vi "Demo_PlotMusic_app.vi"   [LabVIEW 2021, in "RocketPlotDemo.lvlib"]
uses:
  Demo/RocketPlotDemo.lvlib
  Classes/RocketPlotHandle/SubVIs/Init Options.ctl
  TypeDefs/TimeZone.ctl
  TypeDefs/plot load data V2.ctl
  TypeDefs/plot properties V2.ctl
  TypeDefs/plot attributes V2.ctl
  TypeDefs/Plot scale axis properties.ctl
  TypeDefs/Plot general properties.ctl
  <vilib>/sound2/lvsound2.llb/Sampling Mode.ctl
  Classes/RocketPlotPanel/RocketPlotPanel.lvclass/RocketPlotPanel.ctl
  Classes/BjusticePlotHandle/BjusticePlotHandle.lvclass/BjusticePlotHandle.ctl
  4dfea61d-788a-4186-b191-4cde70d6fed2.vi
  966c8643-725a-46bd-9dd0-b91467cf4ddd.vi
  eb0507fd-03f2-4275-8513-22fa9a77d05c.vi
  2cc444ce-eb93-4e53-95b9-bbf802b1ec09.vi
  44d01159-0067-4c41-b020-b8d23d8c44ab.vi
  0323ff41-b8ad-4ed8-8c31-07cadd3001fa.vi
  286f873d-ace6-4cc1-b7d0-d8c3bbebe2d8.vi
  d8c1f50c-a031-4c7b-bbc9-5a9a3e4568ff.vi
  d49b8d8d-7917-4e09-824a-362aaf82a6cf.vi
  35cc1419-e3af-44ec-a6f0-6af3754db062.vi
  Classes/RocketPlotPanel/Read RocketPlotHandle.vi
  Classes/BjusticePlotHandle/Read sub names.vi
  Classes/BjusticePlotHandle/Read time to plot.vi
  <userlib>/bjustice/Ring Buffer for Time Series Data Strict Accessor/Unix time epoch/Unix_Epoch_in_Labview.vi
  44d01159-0067-4c41-b020-b8d23d8c44ab.vi/4c2a6c61-f100-483c-8a49-51e57025a24c.vi
  44d01159-0067-4c41-b020-b8d23d8c44ab.vi/e57bc314-87c7-4952-9bc8-929005dac297.vi
  0323ff41-b8ad-4ed8-8c31-07cadd3001fa.vi/4c2a6c61-f100-483c-8a49-51e57025a24c.vi
  0323ff41-b8ad-4ed8-8c31-07cadd3001fa.vi/e57bc314-87c7-4952-9bc8-929005dac297.vi
  <userlib>/bjustice/Ring Buffer for Time Series Data/API Poly.vi
  <userlib>/bjustice/Ring Buffer for Time Series Data/API/Write Array.vi
  d8c1f50c-a031-4c7b-bbc9-5a9a3e4568ff.vi/f2df9050-0eef-46c6-aff6-3ce3a8893ea5.vi
  35cc1419-e3af-44ec-a6f0-6af3754db062.vi/f2df9050-0eef-46c6-aff6-3ce3a8893ea5.vi
  <userlib>/bjustice/Ring Buffer for Time Series Data/SubVIs/Split Values Array.vi
  <userlib>/bjustice/Ring Buffer for Time Series Data/SubVIs/Replace Values Array Multiple Timestamps.vi
  d8c1f50c-a031-4c7b-bbc9-5a9a3e4568ff.vi/f2df9050-0eef-46c6-aff6-3ce3a8893ea5.vi/63c583a5-c20f-4aba-9c90-661423dee4c4.vi
  d8c1f50c-a031-4c7b-bbc9-5a9a3e4568ff.vi/f2df9050-0eef-46c6-aff6-3ce3a8893ea5.vi/52385341-3d9c-45d2-aff5-e082a4793eb1.vi
  d8c1f50c-a031-4c7b-bbc9-5a9a3e4568ff.vi/f2df9050-0eef-46c6-aff6-3ce3a8893ea5.vi/37f29efa-f142-46b1-a185-f0098a95fbb6.vi
  d8c1f50c-a031-4c7b-bbc9-5a9a3e4568ff.vi/f2df9050-0eef-46c6-aff6-3ce3a8893ea5.vi/84b3d231-9afe-4b6e-afae-e0be43a31e4e.vi
  d8c1f50c-a031-4c7b-bbc9-5a9a3e4568ff.vi/f2df9050-0eef-46c6-aff6-3ce3a8893ea5.vi/c726271c-fc36-4bb7-8553-8945ec40c1cd.vi
  d8c1f50c-a031-4c7b-bbc9-5a9a3e4568ff.vi/f2df9050-0eef-46c6-aff6-3ce3a8893ea5.vi/a7b1d944-dc88-46f5-9d3e-305d46bbe1f6.vi
  d8c1f50c-a031-4c7b-bbc9-5a9a3e4568ff.vi/f2df9050-0eef-46c6-aff6-3ce3a8893ea5.vi/8abc4a6e-a1d2-4e85-879b-517e0ab55733.vi
  d8c1f50c-a031-4c7b-bbc9-5a9a3e4568ff.vi/f2df9050-0eef-46c6-aff6-3ce3a8893ea5.vi/bd347357-b475-4a03-9ac5-3b85ef11aecc.vi
  d8c1f50c-a031-4c7b-bbc9-5a9a3e4568ff.vi/f2df9050-0eef-46c6-aff6-3ce3a8893ea5.vi/391b36e9-a702-45e4-9499-3914f8833a58.vi
  d8c1f50c-a031-4c7b-bbc9-5a9a3e4568ff.vi/f2df9050-0eef-46c6-aff6-3ce3a8893ea5.vi/44155b33-c915-49ce-9e44-a66693aa70dd.vi
  d8c1f50c-a031-4c7b-bbc9-5a9a3e4568ff.vi/f2df9050-0eef-46c6-aff6-3ce3a8893ea5.vi/36977d53-dbe0-4dbc-b2ac-3dea4345b868.vi
  35cc1419-e3af-44ec-a6f0-6af3754db062.vi/f2df9050-0eef-46c6-aff6-3ce3a8893ea5.vi/63c583a5-c20f-4aba-9c90-661423dee4c4.vi
  35cc1419-e3af-44ec-a6f0-6af3754db062.vi/f2df9050-0eef-46c6-aff6-3ce3a8893ea5.vi/52385341-3d9c-45d2-aff5-e082a4793eb1.vi
  35cc1419-e3af-44ec-a6f0-6af3754db062.vi/f2df9050-0eef-46c6-aff6-3ce3a8893ea5.vi/37f29efa-f142-46b1-a185-f0098a95fbb6.vi
  35cc1419-e3af-44ec-a6f0-6af3754db062.vi/f2df9050-0eef-46c6-aff6-3ce3a8893ea5.vi/84b3d231-9afe-4b6e-afae-e0be43a31e4e.vi
  35cc1419-e3af-44ec-a6f0-6af3754db062.vi/f2df9050-0eef-46c6-aff6-3ce3a8893ea5.vi/c726271c-fc36-4bb7-8553-8945ec40c1cd.vi
  35cc1419-e3af-44ec-a6f0-6af3754db062.vi/f2df9050-0eef-46c6-aff6-3ce3a8893ea5.vi/a7b1d944-dc88-46f5-9d3e-305d46bbe1f6.vi
  35cc1419-e3af-44ec-a6f0-6af3754db062.vi/f2df9050-0eef-46c6-aff6-3ce3a8893ea5.vi/8abc4a6e-a1d2-4e85-879b-517e0ab55733.vi
  35cc1419-e3af-44ec-a6f0-6af3754db062.vi/f2df9050-0eef-46c6-aff6-3ce3a8893ea5.vi/bd347357-b475-4a03-9ac5-3b85ef11aecc.vi
  35cc1419-e3af-44ec-a6f0-6af3754db062.vi/f2df9050-0eef-46c6-aff6-3ce3a8893ea5.vi/391b36e9-a702-45e4-9499-3914f8833a58.vi
  35cc1419-e3af-44ec-a6f0-6af3754db062.vi/f2df9050-0eef-46c6-aff6-3ce3a8893ea5.vi/44155b33-c915-49ce-9e44-a66693aa70dd.vi
  35cc1419-e3af-44ec-a6f0-6af3754db062.vi/f2df9050-0eef-46c6-aff6-3ce3a8893ea5.vi/36977d53-dbe0-4dbc-b2ac-3dea4345b868.vi
  <userlib>/bjustice/Ring Buffer for Time Series Data/SubVIs/Enforce array size multiple timestamps.vi
  Classes/BjusticePlotHandle/BjusticePlotHandle.lvclass
  C:/Users/bjustice/Documents/GitHub/BluePlot/Source/Classes/RocketPlotHandle/RocketPlotHandle.lvclass
  Classes/RocketPlotPanel/RocketPlotPanel.lvclass
  C:/Program Files/National Instruments/LabVIEW 2021/vi.lib/IlluminatedG/IG OOPanel/OOPanel/Panel/Panel.lvclass
  <vilib>/sound2/lvsound2.llb/Sound File Info (path).vi
  <vilib>/sound2/lvsound2.llb/Sound File Read Open.vi
  <vilib>/sound2/lvsound2.llb/Sound Output Set Volume (Single).vi
  Classes/RocketPlotHandle/Load PlotConfig.vi
  <vilib>/sound2/lvsound2.llb/Sound File Read (DBL).vi
  <vilib>/Utility/error.llb/Error Cluster From Error Code.vi
  <vilib>/sound2/lvsound2.llb/Sound Output Write (DBL).vi
  Classes/RocketPlotHandle/RocketPlotHandle.lvclass
  RocketPlot.lvlib
  <userlib>/bjustice/Ring Buffer for Time Series Data Strict Accessor/Ring Buffer Strict Accessor.lvlib
  <vilib>/IlluminatedG/IG OOPanel/OOPanel/Manager/Manager.lvclass
  C:/Users/bjustice/Documents/GitHub/BluePlot/Source/Classes/BjusticePlotHandle/BjusticePlotHandle.lvclass
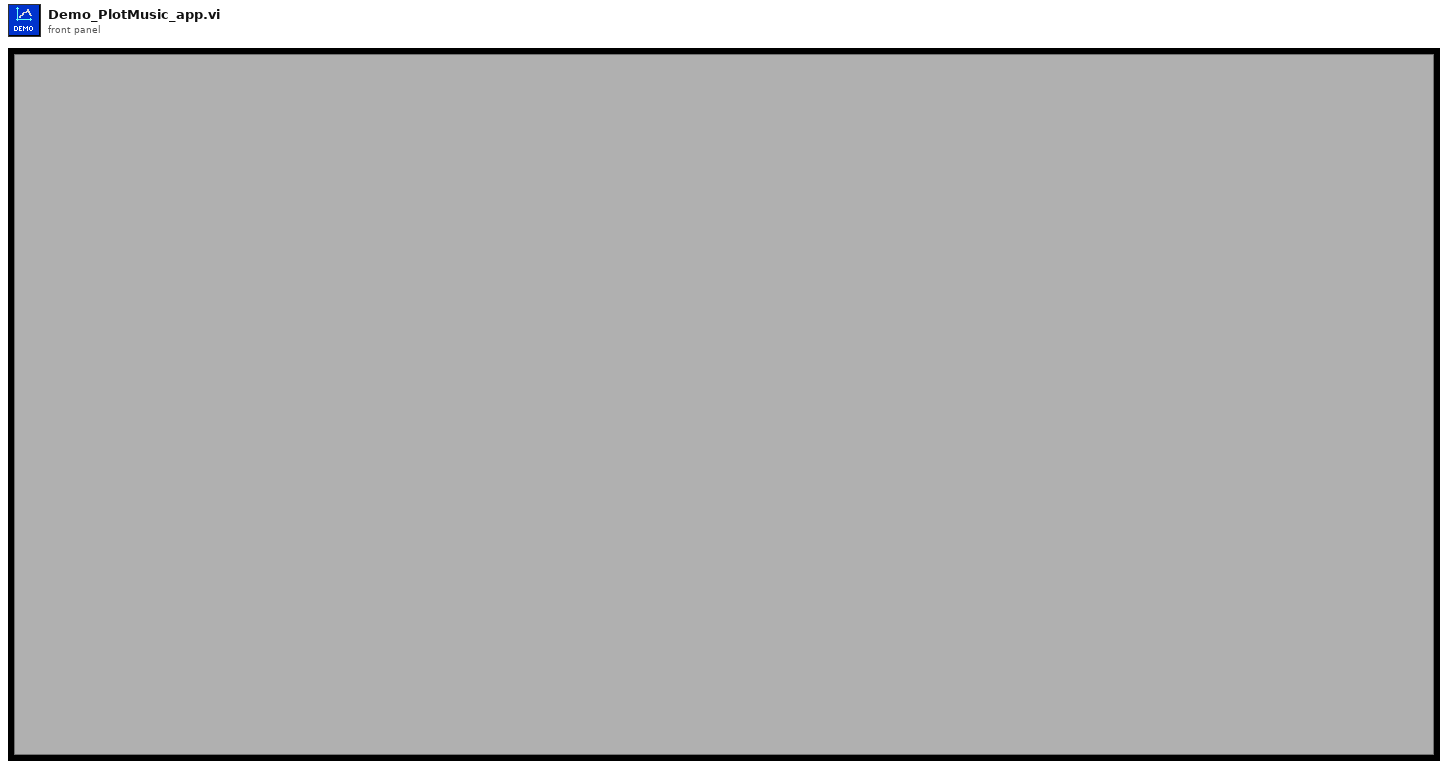
[diagram p1: front panel]
types:
  T1 = typedef "Sampling Mode.ctl" = i32
  T2 = typedef "RocketPlot.lvlib/plot load data V2.ctl" = cluster{"plots":T3[], "X-axis":T5, "Y-axes":T5[], "General":T6}
  T3 = typedef "RocketPlot.lvlib/plot properties V2.ctl" = cluster{"attributes":T4, "Numeric":dbl, "Flatline?":bool}
  T4 = typedef "RocketPlot.lvlib/plot attributes V2.ctl" = cluster{"Plot Color":u32, "Point Style":u8, "Line Style":u8, "Plot Interpolation":u8, "Line Width":u8, "Bar Plot Style":u8, "Fill To":i16, "X Scale Index":u32, "Y Scale Index":u32, "Anti-aliased":bool, "Label Format":u8, "Digital Transition Type":u8, "Digital Transition Location":u8, "Digital Line Style":u8, "Fill/Point Color":u32, "Plot Name":string, "Visible":bool}
  T5 = typedef "RocketPlot.lvlib/Plot scale axis properties.ctl" = cluster{"Name Label.Text":string, "Style":u8, "Tick Colors:Minor Tick Color":u32, "Tick Colors:Tick Color":u32, "Marker Colors:Text Color":u32, "Grid Colors:Major Color":u32, "Grid Colors:Minor Color":u32, "Mapping Mode":u8, "Flipped":bool, "Name Label.Visible":bool, "Name Label.Text Colors:Text Color":u32, "Scale Fit":u8, "Range:Maximum":dbl, "Range:Minimum":dbl, "Offset and Multiplier:Multiplier":dbl, "Offset and Multiplier:Offset":dbl, "Name Label.Font:Size":u32, "Marker.Font:Size":u32, "Uniform Marker Spacing?":bool, "Format String":string}
  T6 = typedef "RocketPlot.lvlib/Plot general properties.ctl" = cluster{"Title":string, "Time to Plot":dbl, "Title.Visible":bool, "Sidebar.Visible":bool, "Plot Area:Colors:BG Color":u32, "X Scale.Plot Name":string, "X Scale.Use Plot Name":bool}
  T7 = typedef "RocketPlotHandle.lvclass/Init Options.ctl" = cluster{"UI visible?":bool, "Update rate (ms)":u32, "Sidebar.Visible":bool, "time to plot (init)":dbl, "time to plot (max)":dbl, "config file start path":path, "Title.Visible":bool, "Title":string, "TimeZone":T8}
  T8 = typedef "RocketPlot.lvlib/TimeZone.ctl" = enum16{"UTC", "Local"}
  T9 = typedef "Sound Data Format.ctl" = cluster{"sample rate (S/s)":dbl, "number of channels":i32, "bits per sample":i32}
  T10 = typedef "Ring Buffer Strict Accessor.lvlib/RingBufferHandle.ctl" = cluster{"Ring buffer DVR":refnum<data-value>, "Data Type":T11, "Size(s)":i32[], "Endianess":T12, "Buffer Size (#timestamps) [init]":i32}
  T11 = typedef "Ring Buffer Strict Accessor.lvlib/DataType.ctl" = enum16{"uint8", "uint16", "uint32", "uint64", "int8", "int16", "int32", "int64", "float", "double", "extended"}
  T12 = typedef "Ring Buffer Strict Accessor.lvlib/Endianess.ctl" = enum16{"big-endian", "little-endian"}
  T13 = typedef "Sound File Refnum.ctl" = refnum<file>
  T14 = typedef "Sound Output Task ID.ctl" = u32
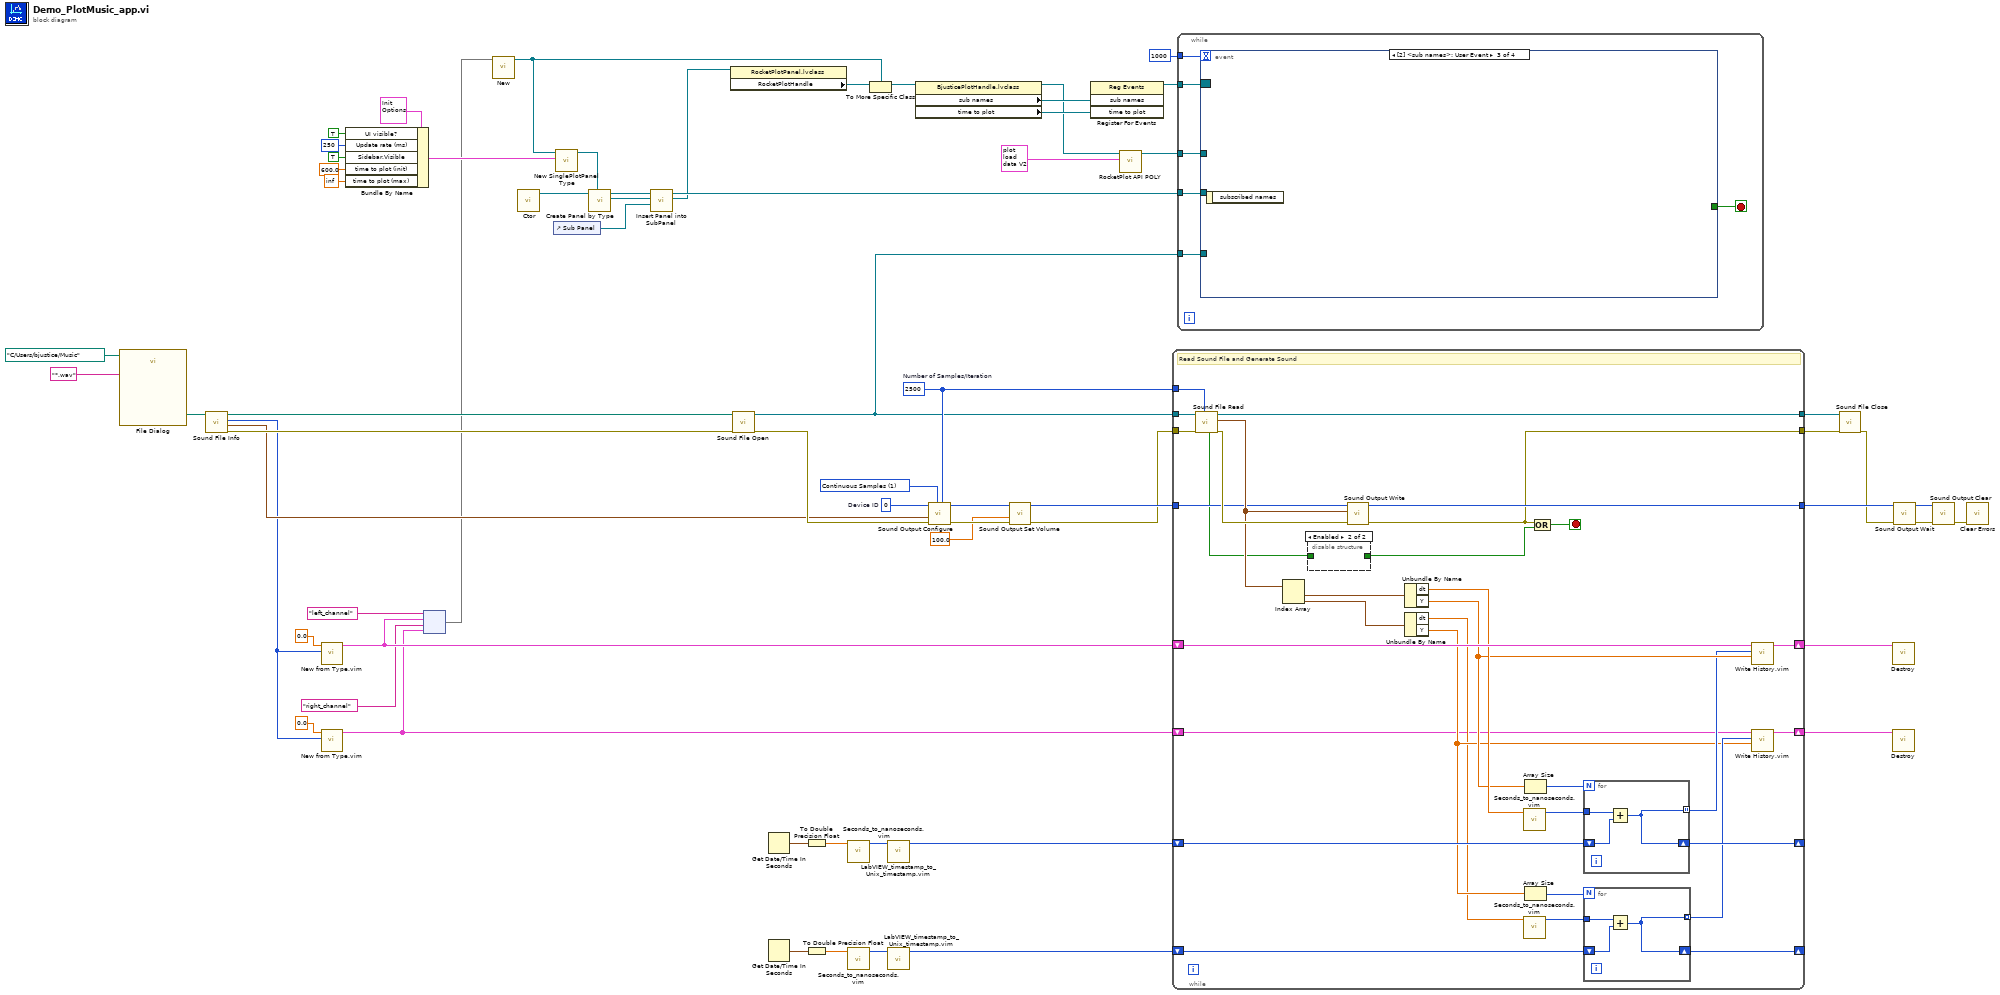
[diagram p0: block diagram]
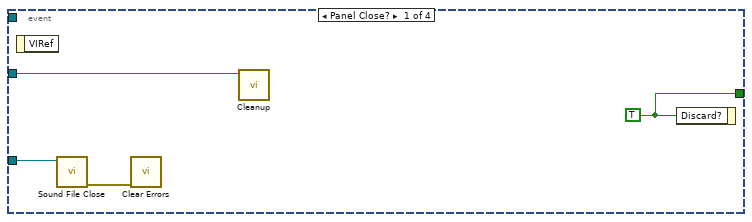
[diagram p2: hidden frame]
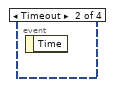
[diagram p3: hidden frame]
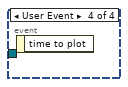
[diagram p4: hidden frame]
diagram:
  w26 = u32 0  # Device ID
  w25 = T1 1 items=["Finite Samples", "Continuous Samples"] ("sample mode")
  w58 = 2500  # Number of Samples/Iteration
  n1 = call "File Dialog"("start path"=path "C:/Users/bjustice/Music" ("path"), "pattern (all files)"="*.wav") -> ("selected path"=w1:path)  [unwired: 10 in, 3 out]
  n2 = call-poly <vilib>:"Sound File Info.vi"("path"=w1) -> ("error out"=w63:errorcluster, "sound format"=w38:T9, "total number of samples/ch"=w28:u32, "path out"=w59:path)  [unwired: 7 in]
  n3 = call "New from Type.vim"("Buffer Size (#timestamps)"=w28, "LV type (array size cannot be empty)"=0.0 ("value")) -> ("Ring Buffer"=w16:T10)  [unwired: 8 in, 1 out]
  n4 = call "New from Type.vim"("Buffer Size (#timestamps)"=w28, "LV type (array size cannot be empty)"=0.0 ("value")) -> ("Ring Buffer"=w14:T10)  [unwired: 8 in, 1 out]
  n5 = Bundle By Name(cluster=T7 {"UI visible?"=TRUE, "Update rate (ms)"=250, "Sidebar.Visible"=TRUE, "time to plot (init)"=600.0, "time to plot (max)"=inf, "config file start path"=path "", "Title.Visible"=TRUE, "Title"="Title", "TimeZone"=enum."Local"} ("Init options"), "UI visible?"=TRUE, "Update rate (ms)"=u32 250, "Sidebar.Visible"=TRUE ("visible sidebar?"), "time to plot (init)"=600.0, "time to plot (max)"=inf) -> (w48:T7)
  n6 = node("left_channel" ("Name (Read/Add)"), w16, "right_channel" ("Name (Read/Add)"), w14) -> (w13:map{string, T10})
  n7 = call <userlib>:"New.vi"("ChannelMap"=w13) -> ("StokePlotHandle out"=w9:refnum<class "BjusticePlotHandle.lvclass">)  [unwired: 9 in, 1 out]
  n8 = call <vilib>:"Ctor.vi"() -> ("Manager out"=w49:refnum<class "Manager.lvclass">)  [unwired: 10 in, 1 out]
  n9 = control-ref of="Sub Panel"() -> (w45:refnum<vi>)
  n10 = call "New SinglePlotPanel Type.vi"("Init options"=w48, "BluePlotHandle"=w9) -> ("SinglePlotPanel out"=w47:refnum<class "RocketPlotPanel.lvclass">)  [unwired: 8 in, 1 out]
  n11 = call <vilib>:"Create Panel by Type.vi"("Panel Type"=w47, "Manager in"=w49) -> ("Panel"=w44:refnum<class "RocketPlotPanel.lvclass">, "Manager out"=w46:refnum<class "Manager.lvclass">)  [unwired: 7 in, 1 out]
  n12 = call <vilib>:"Insert Panel into SubPanel.vi"("SubPanel"=w45, "Panel In"=w44, "Manager in"=w46) -> ("Panel"=w10:refnum<class "RocketPlotPanel.lvclass">, "Manager out"=w43:refnum<class "Manager.lvclass">)  [unwired: 6 in, 1 out]
  n13 = property class="RocketPlotPanel.lvclass"(reference=w10) -> ("RocketPlotHandle"=w12:refnum<class "RocketPlotHandle.lvclass">)  [unwired: 1 in, 2 out]
  n14 = call-poly <vilib>:"Sound File Open.vi"("error in (no error)"=w63, "path"=w59) -> ("error out"=w62:errorcluster, "sound file refnum"=w29:T13)  [unwired: 8 in]
  n15 = Get Date/Time In Seconds() -> (seconds since 1Jan1904=w40:timestamp)
  n16 = Get Date/Time In Seconds() -> (seconds since 1Jan1904=w33:timestamp)
  n17 = To Double Precision Float(number=w40) -> (double precision float=w39:dbl)
  n18 = To Double Precision Float(number=w33) -> (double precision float=w34:dbl)
  n19 = call "Seconds_to_nanoseconds.vim"("timestamp (seconds)"=w39) -> ("timestamp (nanoseconds)"=w42:u64)  [unwired: 10 in]
  n20 = call "Seconds_to_nanoseconds.vim"("timestamp (seconds)"=w34) -> ("timestamp (nanoseconds)"=w32:u64)  [unwired: 10 in]
  n21 = To More Specific Class(target class=w9, reference=w12) -> (specific class reference=w11:refnum<class "BjusticePlotHandle.lvclass">)  [unwired: 1 in, 1 out]
  n22 = call "LabVIEW_timestamp_to_Unix_timestamp.vim"("LabVIEW timestamp (nanoseconds)"=w42) -> ("Unix timestamp (nanoseconds)"=w36:u64)  [unwired: 10 in]
  n23 = call "LabVIEW_timestamp_to_Unix_timestamp.vim"("LabVIEW timestamp (nanoseconds)"=w32) -> ("Unix timestamp (nanoseconds)"=w35:u64)  [unwired: 10 in]
  n24 = property class="BjusticePlotHandle.lvclass"(reference=w11) -> (reference out=w6:refnum<class "BjusticePlotHandle.lvclass">, "sub names"=w8:refnum<user-event>, "time to plot"=w7:refnum<user-event>)  [unwired: 1 in, 1 out]
  n25 = call <vilib>:"Sound Output Configure.vi"("number of samples/ch"=w58, "sample mode"=w25, "error in (no error)"=w62, "sound format"=w38, "device ID"=w26) -> ("error out"=w20:errorcluster, "task ID"=w21:T14)  [unwired: 5 in]
  n26 = call-poly <vilib>:"Sound Output Set Volume.vi"("error in (no error)"=w20, "volume"=100.0, "task ID"=w21) -> ("error out"=w18:errorcluster, "task ID out"=w19:T14)  [unwired: 7 in]
  n27 = register-events(w8, w7) -> (reference out=w5:refnum<event-registration>)  [unwired: 2 in, 1 out]
  n28 = call-poly "RocketPlot API POLY.vi"("Plot config"=T2 {"plots"=[{"attributes"={"Plot Color"=16711680, "Point Style"=0, "Line Style"=0, "Plot Interpolation"=2, "Line Width"=0, "Bar Plot Style"=0, "Fill To"=-1, "X Scale Index"=0, "Y Scale Index"=0, "Anti-aliased"=FALSE, "Label Format"=3, "Digital Transition Type"=0, "Digital Transition Location"=2, "Digital Line Style"=1, "Fill/Point Color"=16711680, "Plot Name"="left_channel", "Visible"=TRUE}, "Numeric"=0.0, "Flatline?"=FALSE}, {"attributes"={"Plot Color"=4387583, "Point Style"=0, "Line Style"=0, "Plot Interpolation"=2, "Line Width"=0, "Bar Plot Style"=0, "Fill To"=-1, "X Scale Index"=0, "Y Scale Index"=1, "Anti-aliased"=FALSE, "Label Format"=3, "Digital Transition Type"=0, "Digital Transition Location"=2, "Digital Line Style"=1, "Fill/Point Color"=4387583, "Plot Name"="right_channel", "Visible"=TRUE}, "Numeric"=0.0, "Flatline?"=FALSE}, {"attributes"={"Plot Color"=16722671, "Point Style"=0, "Line Style"=0, "Plot Interpolation"=2, "Line Width"=5, "Bar Plot Style"=0, "Fill To"=-1, "X Scale Index"=0, "Y Scale Index"=0, "Anti-aliased"=FALSE, "Label Format"=3, "Digital Transition Type"=0, "Digital Transition Location"=2, "Digital Line Style"=1, "Fill/Point Color"=16722671, "Plot Name"="", "Visible"=TRUE}, "Numeric"=0.0, "Flatline?"=FALSE}], "X-axis"={"Name Label.Text"="Time (s)", "Style"=0, "Tick Colors:Minor Tick Color"=16777216, "Tick Colors:Tick Color"=3684408, "Marker Colors:Text Color"=16448250, "Grid Colors:Major Color"=3684408, "Grid Colors:Minor Color"=16777216, "Mapping Mode"=0, "Flipped"=FALSE, "Name Label.Visible"=TRUE, "Name Label.Text Colors:Text Color"=16448250, "Scale Fit"=2, "Range:Maximum"=3867076442.0, "Range:Minimum"=3867076433.0, "Offset and Multiplier:Multiplier"=1.0, "Offset and Multiplier:Offset"=0.0, "Name Label.Font:Size"=15, "Marker.Font:Size"=15, "Uniform Marker Spacing?"=TRUE, "Format String"="%<%H:%M:%S>T"}, "Y-axes"=[{"Name Label.Text"="Left Axis", "Style"=0, "Tick Colors:Minor Tick Color"=16777216, "Tick Colors:Tick Color"=3684408, "Marker Colors:Text Color"=16448250, "Grid Colors:Major Color"=3684408, "Grid Colors:Minor Color"=16777216, "Mapping Mode"=0, "Flipped"=FALSE, "Name Label.Visible"=FALSE, "Name Label.Text Colors:Text Color"=16448250, "Scale Fit"=2, "Range:Maximum"=0.5, "Range:Minimum"=-0.5, "Offset and Multiplier:Multiplier"=1.0, "Offset and Multiplier:Offset"=0.0, "Name Label.Font:Size"=15, "Marker.Font:Size"=15, "Uniform Marker Spacing?"=TRUE, "Format String"="%#_g"}, {"Name Label.Text"="Right Axis", "Style"=0, "Tick Colors:Minor Tick Color"=16777216, "Tick Colors:Tick Color"=3684408, "Marker Colors:Text Color"=16448250, "Grid Colors:Major Color"=3684408, "Grid Colors:Minor Color"=16777216, "Mapping Mode"=0, "Flipped"=FALSE, "Name Label.Visible"=FALSE, "Name Label.Text Colors:Text Color"=16448250, "Scale Fit"=2, "Range:Maximum"=0.5, "Range:Minimum"=-0.6000000000000001, "Offset and Multiplier:Multiplier"=1.0, "Offset and Multiplier:Offset"=0.0, "Name Label.Font:Size"=15, "Marker.Font:Size"=15, "Uniform Marker Spacing?"=TRUE, "Format String"="%#_g"}], "General"={"Title"="Title", "Time to Plot"=600.0, "Title.Visible"=TRUE, "Sidebar.Visible"=TRUE, "Plot Area:Colors:BG Color"=0, "X Scale.Plot Name"="", "X Scale.Use Plot Name"=FALSE}} ("Plot config 2"), "BluePlotHandle in"=w6) -> ("BluePlotHandle out"=w51:refnum<class "BjusticePlotHandle.lvclass">)  [unwired: 8 in, 1 out]
  n29 = while {
    tunnel: w58 -> [w91]
    tunnel: w29 -> [w95]
    tunnel: [w94] -> w65
    tunnel: w18 -> [w96]
    tunnel: [w90] -> w64
    tunnel: [w97] -> w61
    shift-right: [w80] -> _
    shift-left: w36 -> [w82]
    shift-right: [w79] -> _
    shift-left: w35 -> [w77]
    shift-right: [w70] -> w31
    shift-left: w16 -> [w88]
    shift-right: [w69] -> w30
    shift-left: w14 -> [w72]
    tunnel: w19 -> [w68]
    stop <- w92 stop-if-true
    # "Read Sound File and Generate Sound"
    n30 = call-poly <vilib>:"Sound File Read.vi"("number of samples/ch (-1: all)"=w91, "error in (no error)"=w96, "sound file refnum"=w95) -> ("error out"=w93:errorcluster, "data"=w89:waveform(dbl)[], "sound file refnum out"=w94:T13, "end of file?"=w67:bool)  [unwired: 4 in, 1 out]
    n31 = Index Array(array=w89) -> (element #1=w87:waveform(dbl), element #2=w71:waveform(dbl))  [unwired: 2 in]
    n32 = disable-structure shown="Enabled" {
      disable-tunnel: w67 -> [w98 _]
      disable-tunnel: [w98 _] -> w66
      frame Disabled {
      }
      frame Enabled {
      }
    }
    n33 = call-poly <vilib>:"Sound Output Write.vi"("error in (no error)"=w93, "data"=w89, "task ID"=w68) -> ("error out"=w90:errorcluster, "task ID out"=w97:T14)  [unwired: 7 in]
    n34 = Unbundle By Name(w87) -> ("dt"=w86:dbl, "Y"=w85:dbl[])
    n35 = Unbundle By Name(w71) -> ("dt"=w73:dbl, "Y"=w74:dbl[])
    n36 = call "Seconds_to_nanoseconds.vim"("timestamp (seconds)"=w86) -> ("timestamp (nanoseconds)"=w83:u64)  [unwired: 10 in]
    n37 = call "Seconds_to_nanoseconds.vim"("timestamp (seconds)"=w73) -> ("timestamp (nanoseconds)"=w76:u64)  [unwired: 10 in]
    n38 = Array Size(array=w85) -> (size(s)=w84:i32)
    n39 = Array Size(array=w74) -> (size(s)=w75:i32)
    n40 = Compound Arithmetic op=OR(w90, w66) -> (w92:bool)
    n41 = for {
      N: w84 -> [_]
      tunnel: w83 -> [w101]
      shift-right: [w99] -> w80
      shift-left: w82 -> [w100]
      tunnel: [w99] -> w81 mode=indexing
      n42 = Add(x=w101, y=w100) -> (x+y=w99:u64)
    }
    n43 = for {
      N: w75 -> [_]
      tunnel: w76 -> [w104]
      shift-right: [w102] -> w79
      shift-left: w77 -> [w103]
      tunnel: [w102] -> w78 mode=indexing
      n44 = Add(x=w104, y=w103) -> (x+y=w102:u64)
    }
    n45 = call "Write History.vim"("LV DataType"=w85, "Timestamps"=w81, "Ring Buffer"=w88) -> ("Ring Buffer"=w70:T10)  [unwired: 7 in, 1 out]
    n46 = call "Write History.vim"("LV DataType"=w74, "Timestamps"=w78, "Ring Buffer"=w72) -> ("Ring Buffer"=w69:T10)  [unwired: 7 in, 1 out]
  }
  n47 = while {
    tunnel: w51 -> [w110]
    tunnel: 1000 ("period (ms)") -> [w108]
    tunnel: w43 -> [w107]
    tunnel: w29 -> [w106]
    tunnel: w5 -> [w105]
    stop <- w109 stop-if-true
    n48 = event shown="[2] <sub names>: User Event" {
      selector: w105 -> [_ _ _ _]
      dyn-events: _ -> [_ _ _ _]
      timeout: w108 -> [_ _ _ _]
      tunnel: w110 -> [_ _ _ _]
      tunnel: [w114 _ _ _] -> w109
      tunnel: w107 -> [w113 _ _ _]
      tunnel: w106 -> [w112 _ _ _]
      event Panel Close? {
        w114 = TRUE ("Discard?")
        n49 = event-data() -> ()  [unwired: 1 in, 1 out]
        n50 = call <vilib>:"Sound File Close.vi"("sound file refnum"=w112) -> ("error out"=w111:errorcluster)  [unwired: 10 in]
        n51 = call <vilib>:"Clear Errors.vi"("error in (no error)"=w111) -> ()  [unwired: 5 in, 2 out]
        n52 = call <vilib>:"Cleanup.vi"("Manager in"=w113) -> ()  [unwired: 8 in, 3 out]
        n53 = event-data("Discard?"=w114) -> ()  [unwired: 1 in, 1 out]
      }
      event Timeout {
        n54 = event-data() -> ()  [unwired: 1 in, 1 out]
      }
      event User Event {
        n55 = event-data() -> ()  [unwired: 1 in, 1 out]
      }
      event User Event {
        n56 = event-data() -> ()  [unwired: 1 in, 1 out]
      }
    }
  }
  n57 = call <vilib>:"Sound File Close.vi"("error in (no error)"=w64, "sound file refnum"=w65) -> ("error out"=w60:errorcluster)  [unwired: 9 in]
  n58 = call <userlib>:"Destroy.vi"("Ring Buffer"=w31) -> ()  [unwired: 10 in, 1 out]
  n59 = call <userlib>:"Destroy.vi"("Ring Buffer"=w30) -> ()  [unwired: 10 in, 1 out]
  n60 = call <vilib>:"Sound Output Wait.vi"("error in (no error)"=w60, "task ID"=w61) -> ("error out"=w23:errorcluster, "task ID out"=w24:T14)  [unwired: 8 in]
  n61 = call <vilib>:"Sound Output Clear.vi"("error in (no error)"=w23, "task ID"=w24) -> ("error out"=w22:errorcluster)  [unwired: 9 in]
  n62 = call <vilib>:"Clear Errors.vi"("error in (no error)"=w22) -> ()  [unwired: 5 in, 2 out]
